vi "Initialize.vi"(8 "error in (no error)":errorcluster caption="Fehler (Eingang, kein Fehler)", 9 "Node address":i8=-1, 10 "Baud Rate":u16(ring)=4 items=["300", "1200", "2400", "4800", "9600", "19200"], 11 "input refnum":refnum<visa-resource-name> caption="Eingang (Referenz)") -> (0 "error out":errorcluster caption="Fehler (Ausgang)", 3 "VISA resource out":refnum<visa-resource-name>)   [LabVIEW 2013, in "Maxi Gauge.lvlib"]
uses:
  <instrlib>/Maxi Gauge/Maxi Gauge.lvlib
panel:
  out "Def. Value":u16=3
  in  "Max Value":u16=5
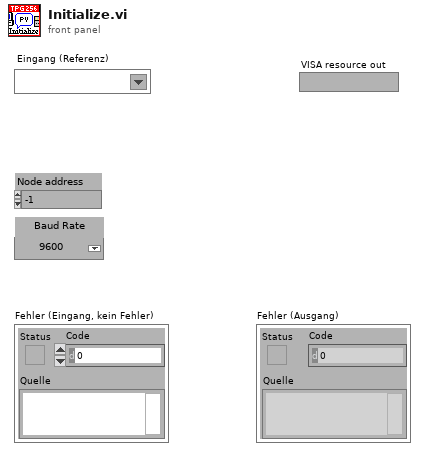
[diagram p1: front panel]
types:
  T1 = enum16{"Init & Test", "Next Baud Rate", "Set Default ", "Communication OK", "Error Box"}
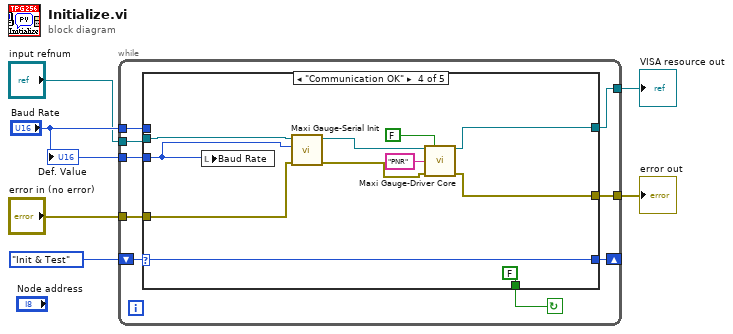
[diagram p0: block diagram]
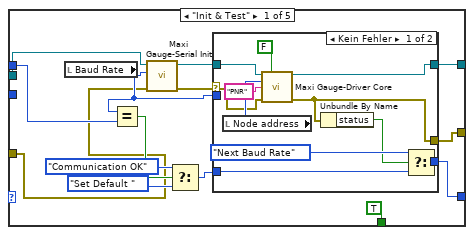
[diagram p2: hidden frame]
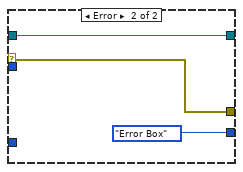
[diagram p3: hidden frame]
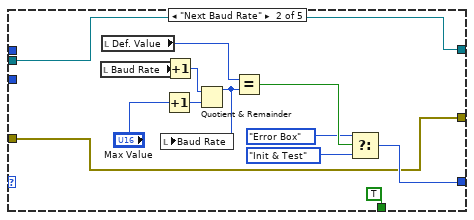
[diagram p4: hidden frame]
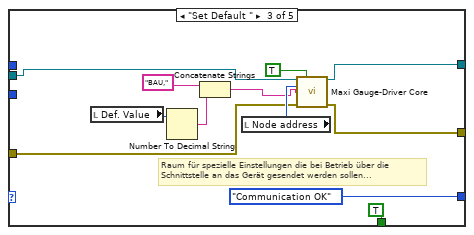
[diagram p5: hidden frame]
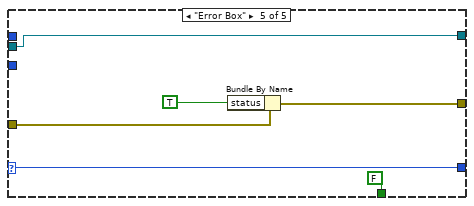
[diagram p6: hidden frame]
diagram:
  n1 = while {
    tunnel: "Baud Rate" -> [w11]
    tunnel: "Baud Rate" -> [w15]
    shift-left: T1."Init & Test" -> [w14]
    shift-right: [w12] -> _
    tunnel: "input refnum" -> [w10]
    tunnel: "error in (no error)" -> [w9]
    tunnel: [w8] -> w2
    tunnel: [w7] -> w1
    stop <- w13 continue-if-true
    n2 = case shown="\"Communication OK\"" w14 {
      selector: w14 -> [_ _ _ w78 w84]
      tunnel: w15 -> [w28 _ _ _ _]
      tunnel: [TRUE TRUE TRUE FALSE FALSE] -> w13
      tunnel: [w23 w47 T1."Communication OK" w78 w84] -> w12
      tunnel: w11 -> [_ _ _ w76 _]
      tunnel: w10 -> [w21 w44 w60 w77 w81]
      tunnel: w9 -> [w19 w45 w58 w75 w83]
      tunnel: [w18 w45 w57 w69 w82] -> w8
      tunnel: [w16 w44 w59 w71 w81] -> w7
      frame "Init & Test" {
        n3 = local read "Baud Rate"() -> (w20:u16)
        n4 = Equal?(x=w20, y=w28) -> (x = y?=w27:bool)
        n5 = call <instrlib>:"Maxi Gauge-Serial Init.vi"("error in (no error)"=w19, "Baud Rate"=w20, "input refnum"=w21) -> ("error out"=w29:errorcluster, "VISA resource out"=w17:refnum<visa-resource-name>)  [unwired: 7 in]
        n6 = Select(t=T1."Communication OK", s=w27, f=T1."Set Default ") -> (s? t:f=w26:T1)
        n7 = case shown="Kein Fehler" w29 {
          selector: w29 -> [w32 w42]
          tunnel: [w40 T1."Error Box"] -> w23
          tunnel: w26 -> [w38 _]
          tunnel: w20 -> [_ _]
          tunnel: [w31 w42] -> w18
          tunnel: w17 -> [w34 w41]
          tunnel: [w33 w41] -> w16
          frame No Error {
            n8 = local read "Node address"() -> (w36:i8)
            n9 = call <instrlib>:"Maxi Gauge-Driver Core.vi"("VISA-Ressource in"=w34, "Write/Read"=FALSE, "Node address"=w36, "Command"="PNR", "Fehler (Eingang)"=w32) -> ("VISA-Ressource out"=w33:refnum<visa-resource-name>, "Fehler (Ausgang)"=w31:errorcluster)  [unwired: 8 in, 1 out]
            n10 = Unbundle By Name(w31) -> ("status"=w30:bool)
            n11 = Select(t=T1."Next Baud Rate", s=w30, f=w38) -> (s? t:f=w40:T1)
          }
          frame Error {
          }
        }
      }
      frame "Next Baud Rate" {
        n12 = local read "Baud Rate"() -> (w46:u16)
        n13 = local read "Def. Value"() -> (w53:u16)
        n14 = Increment(x="Max Value") -> (x+1=w54:u16)
        n15 = Increment(x=w46) -> (x+1=w56:u16)
        n16 = Quotient & Remainder(x=w56, y=w54) -> (x-y*floor(x/y)=w52:u16)  [unwired: 1 out]
        n17 = local write "Baud Rate"(w52) -> ()
        n18 = Equal?(x=w53, y=w52) -> (x = y?=w51:bool)
        n19 = Select(t=T1."Error Box", s=w51, f=T1."Init & Test") -> (s? t:f=w47:T1)
      }
      frame "Set Default " {
        # "Raum für spezielle Einstellungen die bei Betrieb über die\nSchnittstelle an das Gerät gesendet werden sollen..."
        n20 = local read "Def. Value"() -> (w64:u16)
        n21 = Number To Decimal String(number=w64) -> (decimal integer string=w63:string)  [unwired: 1 in]
        n22 = Concatenate Strings("BAU,", w63) -> (w61:string)
        n23 = local read "Node address"() -> (w62:i8)
        n24 = call <instrlib>:"Maxi Gauge-Driver Core.vi"("VISA-Ressource in"=w60, "Write/Read"=TRUE, "Node address"=w62, "Command"=w61, "Fehler (Eingang)"=w58) -> ("VISA-Ressource out"=w59:refnum<visa-resource-name>, "Fehler (Ausgang)"=w57:errorcluster)  [unwired: 8 in, 1 out]
      }
      frame "Communication OK" {
        n25 = local write "Baud Rate"(w76) -> ()
        n26 = call <instrlib>:"Maxi Gauge-Serial Init.vi"("error in (no error)"=w75, "Baud Rate"=w76, "input refnum"=w77) -> ("error out"=w70:errorcluster, "VISA resource out"=w72:refnum<visa-resource-name>)  [unwired: 7 in]
        n27 = call <instrlib>:"Maxi Gauge-Driver Core.vi"("VISA-Ressource in"=w72, "Write/Read"=FALSE, "Command"="PNR", "Fehler (Eingang)"=w70) -> ("VISA-Ressource out"=w71:refnum<visa-resource-name>, "Fehler (Ausgang)"=w69:errorcluster)  [unwired: 9 in, 1 out]
      }
      frame "Error Box" {
        n28 = Bundle By Name(cluster=w83, "status"=TRUE) -> (w82:errorcluster)
      }
    }
  }
  "error out" <- w2
  "VISA resource out" <- w1
  "Def. Value" <- "Baud Rate"
